vi "QScope.vi"() -> ()   [LabVIEW 2018]
uses:
  <vilib>/Utility/miscctls.llb/LVStringsAndValuesArrayTypeDef_DBL.ctl
  <vilib>/express/express signal manip/GetorSetDDTAttributes/Shared VIs/XDimension.ctl
  <vilib>/express/express signal manip/GetorSetDDTAttributes/Shared VIs/TimeType.ctl
  <vilib>/DAQmx/write.llb/DAQmx Write (Analog 1D DBL NChan 1Samp).vi
  <vilib>/DAQmx/read.llb/DAQmx Read (Analog 2D DBL NChan NSamp).vi
  <vilib>/DAQmx/miscellaneous.llb/DAQmx Fill In Error Info.vi
  <vilib>/express/express shared/transition.llb/Dynamic To Waveform Array.vi
  <vilib>/express/express signal manip/GetorSetDDTAttributes/Shared VIs/XDimension Enum to String.vi
  <vilib>/express/express signal manip/GetorSetDDTAttributes/Shared VIs/TimeMode Enum to Boolean.vi
  <vilib>/express/express signal manip/GetorSetDDTAttributes/Set DDT Attributes/SetT0.vi
  <vilib>/express/express signal manip/GetorSetDDTAttributes/Set DDT Attributes/sub Set StartTimeStamp.vi
  <vilib>/express/express shared/transition.llb/Waveform Array To Dynamic.vi
  <vilib>/express/express signal manip/GetorSetDDTAttributes/Get DDT Attributes/Get DDT Properties.xnode
  <vilib>/express/express signal manip/GetorSetDDTAttributes/Set DDT Attributes/Set DDT Properties.xnode
  <resource>/objmgr/daqmx.rc
  <vilib>/express/express signal manip/GetorSetDDTAttributes/Shared VIs/GetSetShared.lvlib
  <vilib>/express/express signal manip/GetorSetDDTAttributes/Set DDT Attributes/Set DDT Attributes.lvlib
panel:
  in  "trace display":enum32{"Time traces", "I-V plot", "Spectrum"}(tab)
  in  "Show \nrecord":i32 min=-1
  out "data":dbl[](graph) caption="Short Trace"
  out "data 2":dbl[](graph) caption="Full Trace"
  in  "Time slide":cluster{dbl, dbl}(slide) scale=0.0..100.0 scale format="%#_3g%"
  in  "short Channel":i8(ring) caption="Channel" items=["Dev2/ai0"]
  in  "long Channel":i8(ring) caption="Channel" items=["Dev2/ai0"]
  in  "fitting\nmethod":i32(ring)=1 items=["nearest", "linear", "spline"]
  out "Record\nTime":string caption="Comment"
  in  "refresh xy-plot":bool caption="Refresh"
  in  "y-channel":u16(ring) items=["Dev2/ai0"]
  in  "x-channel":u16(ring) items=["Dev2/ai0"]
  out "XY Graph":cluster{dbl[], dbl[]}(graph)
  out "time trace":cluster{"X":dbl, "Y":dbl}[](graph)
  out "Frequency domain":cluster{"X":dbl, "Y":dbl}[](graph)
  out "Spectrum":dbl[][](graph)
  in  "File tab":enum32{"File Operations"}(tab)
  in  "Comment\n(25 chars)":string
  out "mean values":dbl[](array[numeric])
  in  "Save to Path":path
  out "Last #":i32
  in  "File name prefix":string="ExpRec-"
  in  "Set threshold?":bool
  in  "Threshold":dbl min=0.0 max=20.0 format="%#_6p"
  out "min values":dbl[](array[numeric])
  out "max values":dbl[](array[numeric])
  out "standard deviation":dbl[](array[numeric])
  in  "Record data":bool
  out "TimeStamp":timestamp format="%<%I:%M:%S %p %d/%m/%Y>T"
  out "file operation error status":errorcluster caption="error out"
  out "Saving Data":bool
  out "active?":bool
  in  "DAQ control":enum32{"DAQ operation", "Analog Output"}(tab)
  in  "Tab Control":enum32{"Input", "Output"}(tab)
  in  "Input Channel List":i32[](listbox)
  in  "Term. Config.":i32(ring)=10083 items=["default"=-1, "RSE"=10083, "NRSE"=10078, "Differential"=10106, "Pseudodifferential"=12529]
  in  "section (s)":dbl=0.1 min=0.1 max=0.6 step=0.1 format="%#.2f"
  in  "full len(s)":dbl=10.0 min=0.5 max=60.0 step=0.5
  in  "Sampling rate (Hz)":dbl=5000.0
  in  "Output Channel List":i32[](listbox)
  in  "output values":dbl[](array[numeric]) format="%0.2f"
  in  "Init Channels":bool
  in  "stop":bool
  out "Recording in progress":bool
  in  "quit":bool
  out "mainloop error status":errorcluster
  out "DAQ error status":errorcluster
  out "DAQTask":refnum<k21>[](array[refnum])
  # "QingLAB@ASU\nhttps://qinglab.physics.edu.asu"
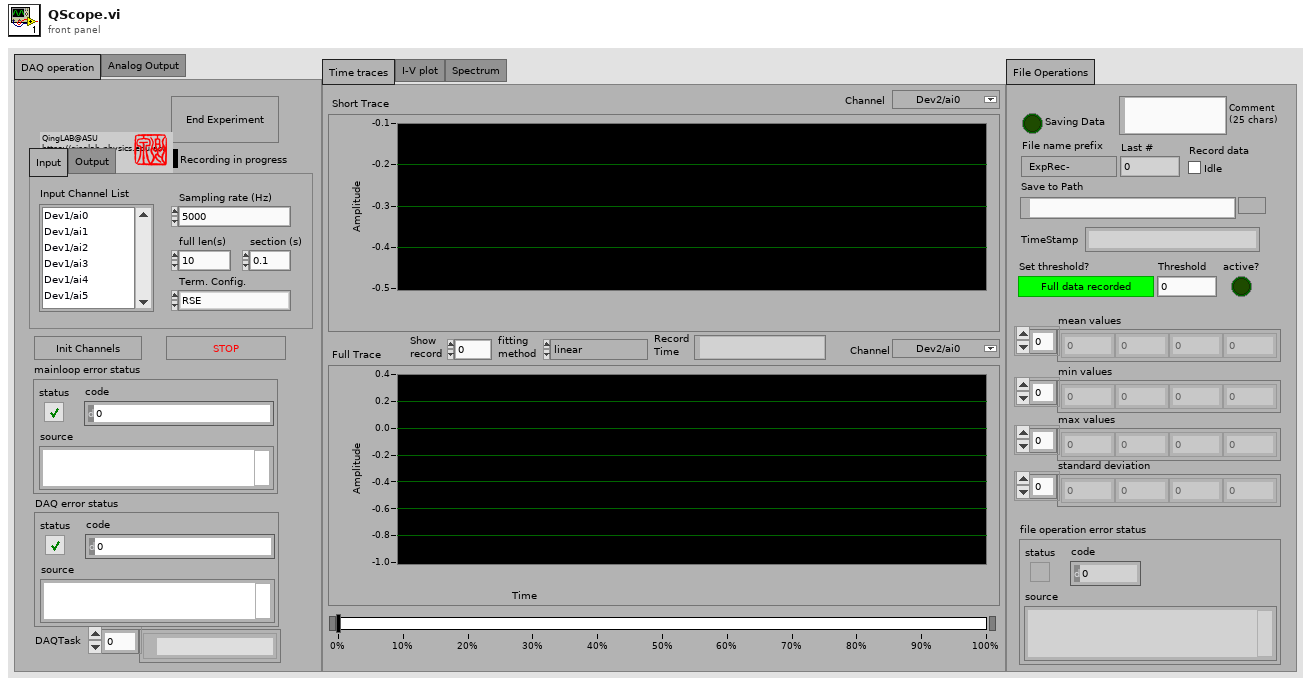
[diagram p1: front panel]
types:
  T1 = enum8{"Enabled", "Disabled", "Disabled and Grayed Out"}
  T2 = typedef "LVStringsAndValuesArrayTypeDef_DBL.ctl" = cluster{"String":string, "Value":dbl}[]
  T3 = cluster{i32, "task out":refnum<k21>[], "data":dbl[][]}
  T4 = typedef "GetSetShared.lvlib/TimeType.ctl" = enum16{"Absolute", "Relative"}
  T5 = typedef "GetSetShared.lvlib/XDimension.ctl" = enum16{"No Unit [-]", "Time [sec]", "Frequency [Hz]"}
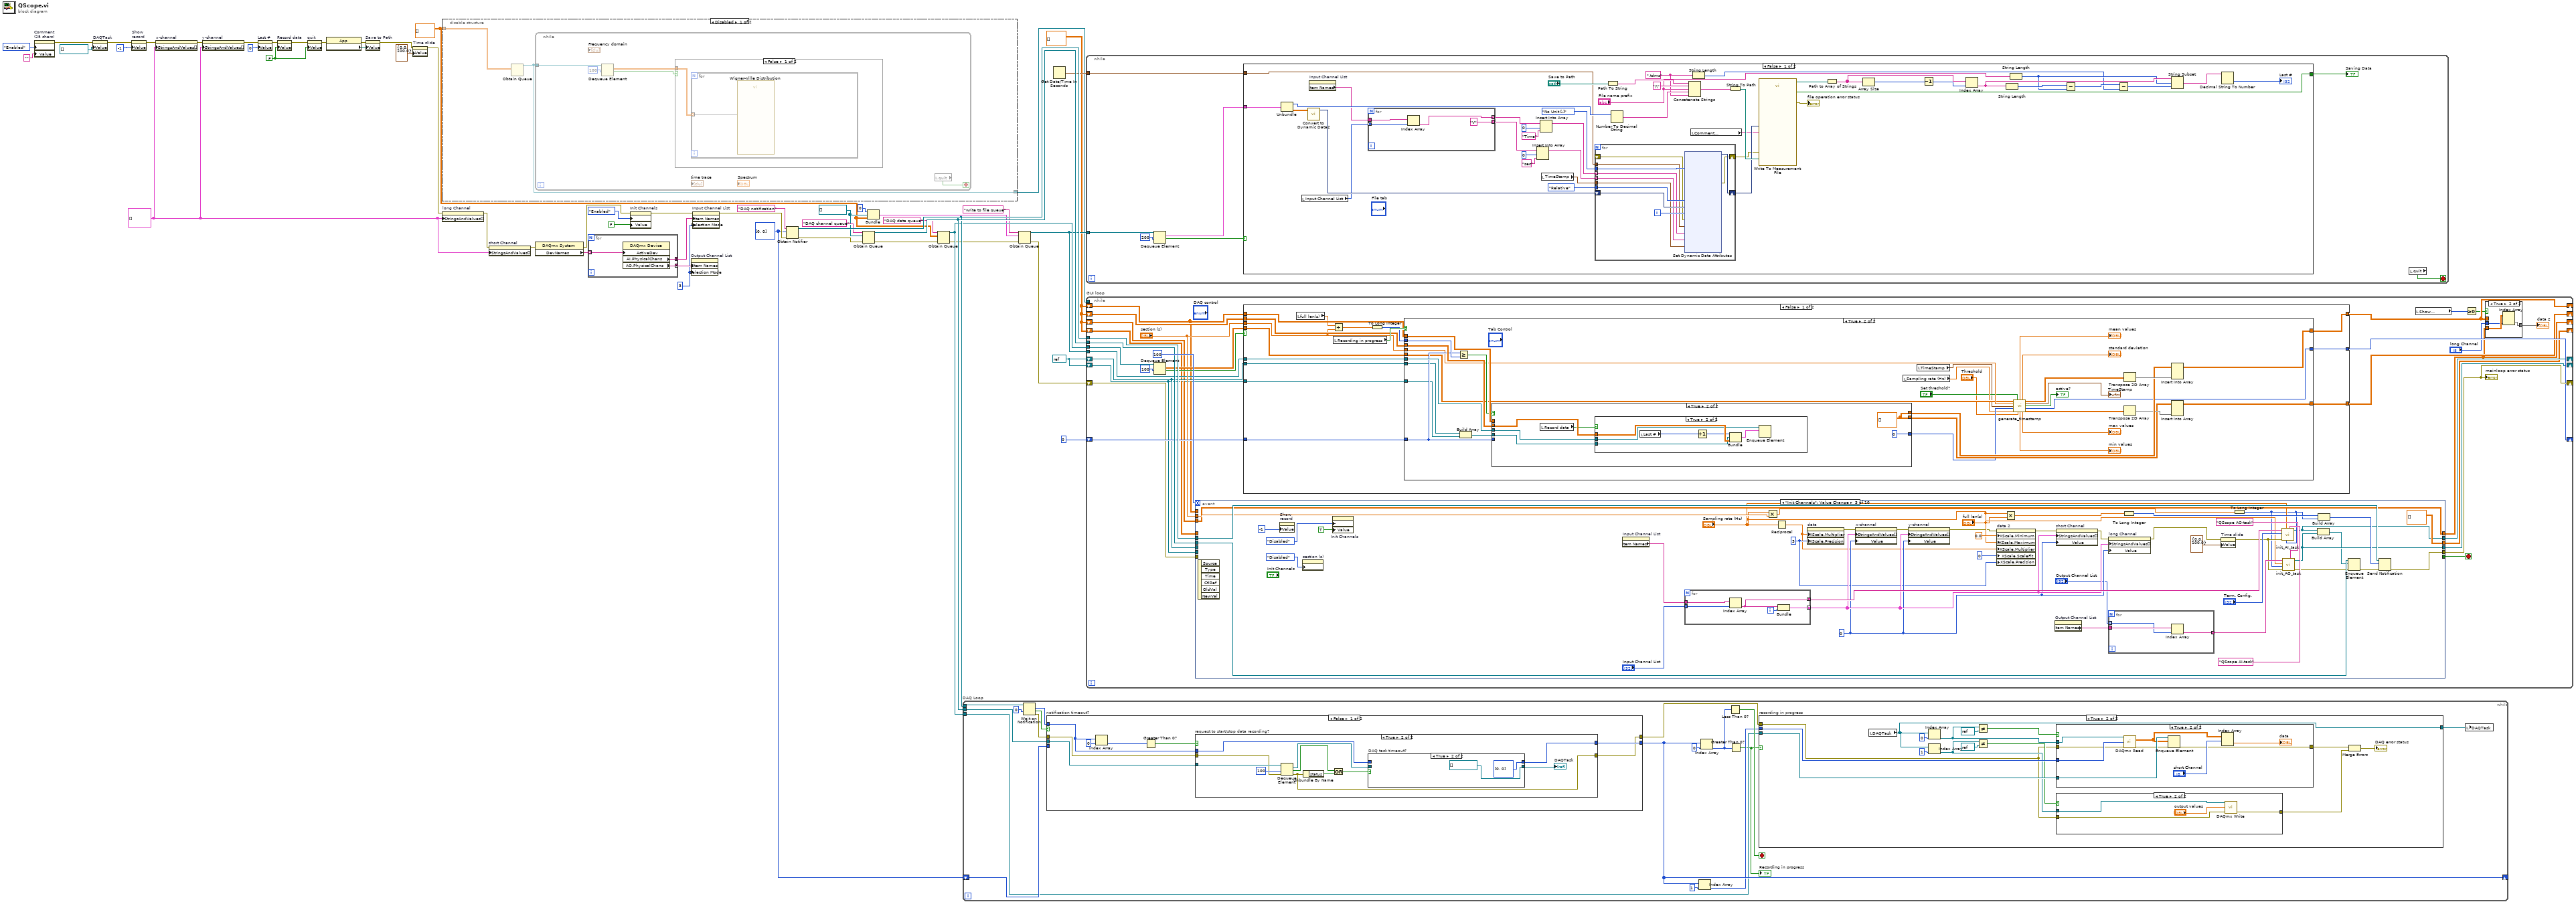
[diagram p0: block diagram]
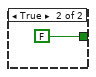
[diagram p4: hidden frame]
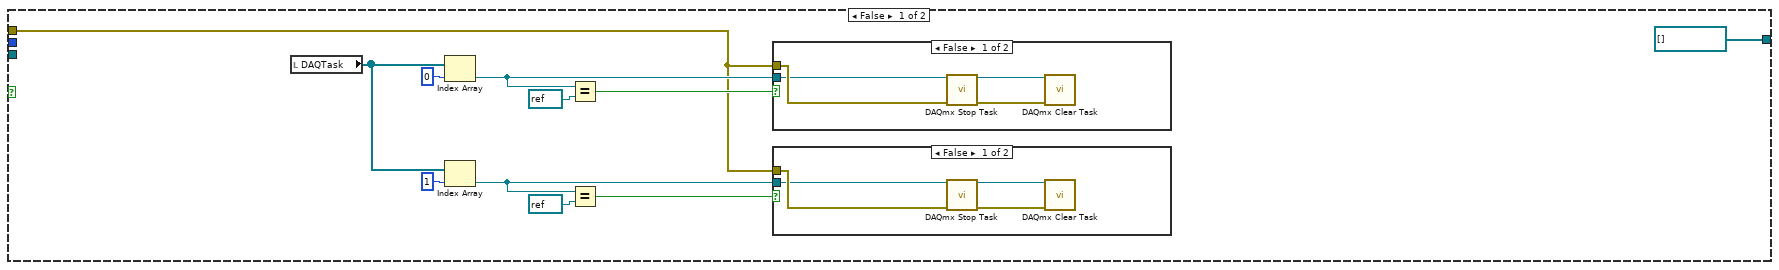
[diagram p5: hidden frame]
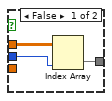
[diagram p13: hidden frame]
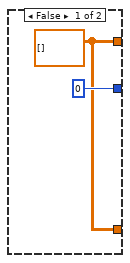
[diagram p14: hidden frame]
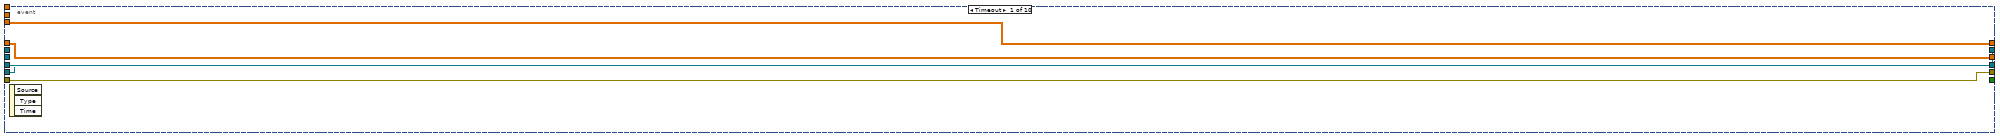
[diagram p18: hidden frame]
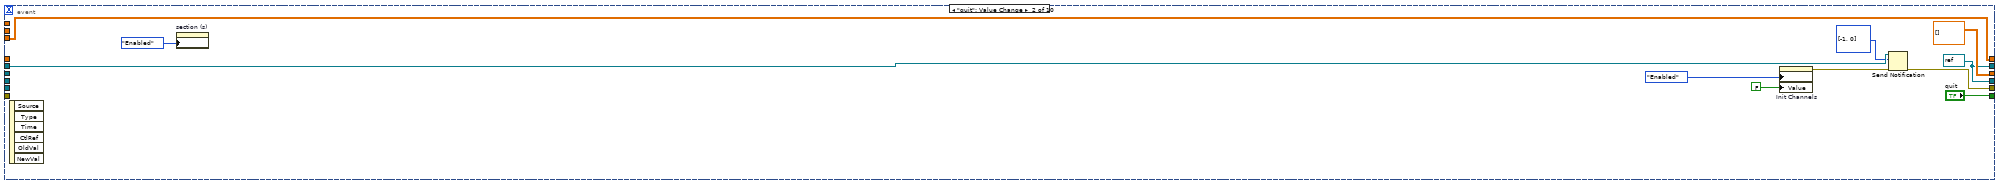
[diagram p19: hidden frame]
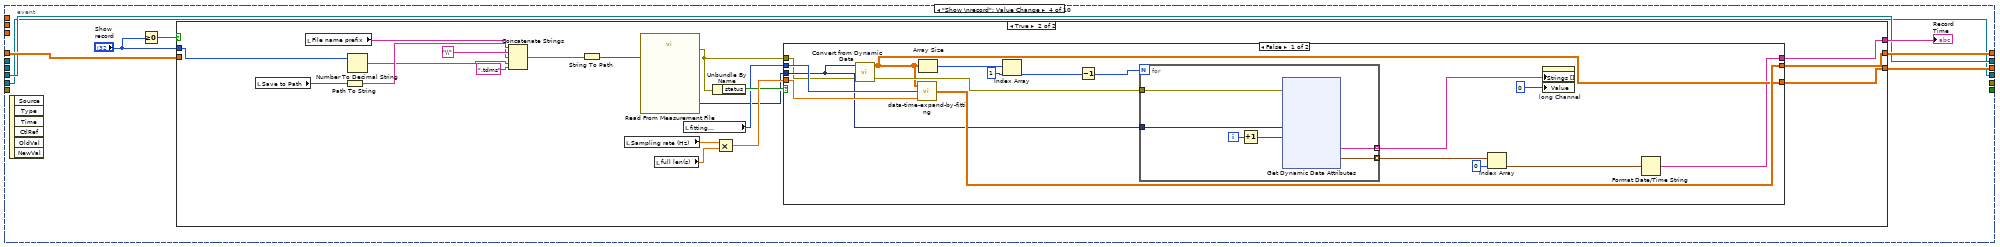
[diagram p20: hidden frame]
diagram:
  w21 = FALSE ("quit")
  w2 = refnum<k21> refnum ("task out")
  w10 = dbl[][] []
  w6 = dbl[][] [] ("data")
  w17 = T2 [] ("Strings And Values []")
  w44 = i32[] [0, 0]
  w25 = refnum<k21>[] [] ("task out")
  w3 = 3 ("Selection Mode")
  n1 = property on="Comment\n(25 chars)" class="Str"("DisabledEnum"=T1."Enabled" ("Disabled"), "Value"="" ("Comment\n(25 chars)")) -> (error out=w7:errorcluster)  [unwired: 2 in, 1 out]
  n2 = property on="DAQTask" class="Arr (strict)"(error in=w7, "Value"=refnum<k21>[] [] ("task out")) -> (error out=w11:errorcluster)  [unwired: 1 in, 1 out]
  n3 = property on="Show \nrecord" class="DigNum (strict)"(error in=w11, "Value"=-1 ("Show previous record")) -> (error out=w12:errorcluster)  [unwired: 1 in, 1 out]
  n4 = property on="x-channel" class="Ring (strict)"(error in=w12, "StringsAndValues[]"=w17) -> (error out=w16:errorcluster)  [unwired: 1 in, 1 out]
  n5 = property on="y-channel" class="Ring (strict)"(error in=w16, "StringsAndValues[]"=w17) -> (error out=w15:errorcluster)  [unwired: 1 in, 1 out]
  n6 = property on="Last #" class="DigNum (strict)"(error in=w15, "Value"=0 ("Last #")) -> (error out=w18:errorcluster)  [unwired: 1 in, 1 out]
  n7 = property on="Record data" class="Bool (strict)"(error in=w18, "Value"=w21) -> (error out=w20:errorcluster)  [unwired: 1 in, 1 out]
  n8 = property on="quit" class="Bool (strict)"(error in=w20, "Value"=w21) -> (error out=w22:errorcluster)  [unwired: 1 in, 1 out]
  n9 = property class="App"(error in=w22) -> (error out=w31:errorcluster, "App.DefaultDataLocation"=w32:path)  [unwired: 1 in, 1 out]
  n10 = property on="Save to Path" class="Path"(error in=w31, "Value"=w32) -> (error out=w30:errorcluster)  [unwired: 1 in, 1 out]
  n11 = property on="Time slide" class="Slide (strict)"(error in=w30, "Value"=cluster{dbl, dbl} {0.0, 100.0} ("Time slide")) -> (error out=w33:errorcluster)  [unwired: 1 in, 1 out]
  n12 = disable-structure shown="Disabled" {
    disable-tunnel: w6 -> [w55 _]
    disable-tunnel: [w54 _] -> w5
    frame Disabled {
      n13 = Obtain Queue(element data type=w55) -> (queue out=w54:refnum<queue>)  [unwired: 4 in, 2 out]
      n14 = while {
        tunnel: w54 -> [w59]
        stop <- w60 stop-if-true
        n15 = Dequeue Element(queue=w59, timeout in ms (-1)=100) -> (element=w56:dbl[][], timed out?=w57:bool)  [unwired: 1 in, 2 out]
        n16 = case shown="False" w57 {
          tunnel: w56 -> [w61 _]
          frame False {
            n17 = for {
              tunnel: w61 -> [w62] mode=indexing
              n18 = call "Wigner-Ville Distribution"("Signal"=w62) -> ()  [unwired: 6 in, 5 out]
            }
          }
          frame True {
          }
        }
        n19 = local read "quit"() -> (w60:bool)
      }
    }
    frame Enabled {
    }
  }
  n20 = property on="long Channel" class="Ring (strict)"(error in=w33, "StringsAndValues[]"=w17) -> (error out=w41:errorcluster)  [unwired: 1 in, 1 out]
  n21 = property on="short Channel" class="Ring (strict)"(error in=w41, "StringsAndValues[]"=w17) -> (error out=w42:errorcluster)  [unwired: 1 in, 1 out]
  n22 = property class="DAQmx System"(error in=w42) -> (error out=w43:errorcluster, "DevNames"=w53:tag[])  [unwired: 1 in, 1 out]
  n23 = for {
    tunnel: w53 -> [w65] mode=indexing
    tunnel: [w64] -> w52 mode=concatenating
    tunnel: [w63] -> w4 mode=concatenating
    n24 = property class="DAQmx Device"("ActiveDev"=w65) -> ("AI.PhysicalChans"=w64:tag[], "AO.PhysicalChans"=w63:tag[])  [unwired: 2 in, 2 out]
  }
  n25 = property on="Init Channels" class="Bool (strict)"(error in=w43, "DisabledEnum"=T1."Enabled" ("Disabled"), "Value"=FALSE ("Init Channels")) -> (error out=w46:errorcluster)  [unwired: 1 in, 1 out]
  n26 = property on="Output Channel List" class="LstBox (strict)"("Item Names"=w4, "Selection Mode"=w3) -> ()  [unwired: 2 in, 2 out]
  n27 = property on="Input Channel List" class="LstBox (strict)"(error in=w46, "Item Names"=w52, "Selection Mode"=w3) -> (error out=w47:errorcluster)  [unwired: 1 in, 1 out]
  n28 = Obtain Notifier(name (unnamed)="DAQ notification", notification data type=w44, error in (no error)=w47) -> (notifier out=w49:refnum<notifier>, error out=w48:errorcluster)  [unwired: 1 in, 1 out]
  n29 = Obtain Queue(name (unnamed)="DAQ channel queue", element data type=w25, error in (no error)=w48) -> (queue out=w50:refnum<queue>, error out=w37:errorcluster)  [unwired: 2 in, 1 out]
  n30 = Bundle(0, "task out"=w25, "data"=w6) -> (w24:T3)  [unwired: 1 in]
  n31 = Obtain Queue(name (unnamed)="DAQ data queue", element data type=w6, error in (no error)=w37) -> (queue out=w36:refnum<queue>, error out=w29:errorcluster)  [unwired: 2 in, 1 out]
  n32 = while "DAQ Loop" {
    tunnel: w50 -> [w78]
    tunnel: w49 -> [w81]
    shift-right: [w71] -> _
    shift-left: w44 -> [w76]
    tunnel: w36 -> [w69]
    stop <- w75 stop-if-true
    n33 = Wait on Notification(notifier=w81, timeout in ms (-1)=0) -> (notification=w79:i32[], timed out?=w80:bool, error out=w77:errorcluster)  [unwired: 2 in, 1 out]
    n34 = case "notification timeout?" shown="False" w80 {
      tunnel: w79 -> [w135 _]
      tunnel: w78 -> [w139 _]
      tunnel: w77 -> [w138 w157]
      tunnel: [w137 w158] -> w71
      tunnel: w76 -> [_ w158]
      tunnel: [w132 w157] -> w68
      frame False {
        n35 = Index Array(array=w135, index=0) -> (element=w133:i32)
        n36 = Greater Than 0?(x=w133) -> (x > 0?=w136:bool)
        n37 = case "request to start/stop data recording?" shown="True" w136 {
          tunnel: w139 -> [_ w152]
          tunnel: w138 -> [w140 w149]
          tunnel: [w141 w148] -> w137
          tunnel: w135 -> [w141 w147]
          tunnel: [w140 w146] -> w132
          frame False {
          }
          frame True {
            n38 = Dequeue Element(queue=w152, timeout in ms (-1)=100, error in (no error)=w149) -> (element=w150:refnum<k21>[], timed out?=w145:bool, error out=w146:errorcluster)  [unwired: 1 out]
            n39 = Unbundle By Name(w146) -> ("status"=w144:bool)
            n40 = Or(x=w145, y=w144) -> (x .or. y?=w143:bool)
            n41 = case "DAQ task timeout?" shown="True" w143 {
              tunnel: w150 -> [w154 _]
              tunnel: [w154 refnum<k21>[] [] ("task out")] -> w142
              tunnel: [w153 i32[] [0, 0]] -> w148
              tunnel: w147 -> [w153 _]
              frame False {
              }
              frame True {
              }
            }
            "DAQTask" <- w142
          }
        }
      }
      frame True {
      }
    }
    n42 = Index Array(array=w71, index=1) -> (element=w70:i32)
    n43 = Index Array(array=w71, index=0) -> (element=w73:i32)
    n44 = Less Than 0?(x=w73) -> (x < 0?=w75:bool)
    n45 = Greater Than 0?(x=w73) -> (x > 0?=w67:bool)
    "Recording in progress" <- w67
    n46 = case "recording in progress" shown="True" w67 {
      tunnel: w70 -> [_ w116]
      tunnel: w69 -> [_ w115]
      tunnel: w68 -> [w84 w106]
      tunnel: [refnum<k21>[] [] ("task out") w102] -> w66
      frame False {
        n47 = local read "DAQTask"() -> (w91:refnum<k21>[])
        n48 = Index Array(array=w91, index=0) -> (element=w88:refnum<k21>)
        n49 = Index Array(array=w91, index=1) -> (element=w85:refnum<k21>)
        n50 = Equal?(x=w88, y=refnum<k21> refnum ("task out")) -> (x = y?=w93:bool)
        n51 = Equal?(x=w85, y=refnum<k21> refnum ("task out")) -> (x = y?=w87:bool)
        n52 = case shown="False" w93 {
          tunnel: w84 -> [w99 _]
          tunnel: w88 -> [w98 _]
          frame False {
            n53 = call <vilib>:"DAQmx Stop Task.vi"("task/channels in"=w98, "error in"=w99) -> ("task out"=w101:refnum<k21>, "error out"=w100:errorcluster)  [unwired: 12 in]
            n54 = call <vilib>:"DAQmx Clear Task.vi"("task in"=w101, "error in"=w100) -> ()  [unwired: 13 in, 1 out]
          }
          frame True {
          }
        }
        n55 = case shown="False" w87 {
          tunnel: w84 -> [w95 _]
          tunnel: w85 -> [w94 _]
          frame False {
            n56 = call <vilib>:"DAQmx Stop Task.vi"("task/channels in"=w94, "error in"=w95) -> ("task out"=w97:refnum<k21>, "error out"=w96:errorcluster)  [unwired: 12 in]
            n57 = call <vilib>:"DAQmx Clear Task.vi"("task in"=w97, "error in"=w96) -> ()  [unwired: 13 in, 1 out]
          }
          frame True {
          }
        }
      }
      frame True {
        n58 = local read "DAQTask"() -> (w102:refnum<k21>[])
        n59 = Index Array(array=w102, index=0) -> (element=w111:refnum<k21>)
        n60 = Index Array(array=w102, index=1) -> (element=w107:refnum<k21>)
        n61 = Not Equal?(x=w111, y=refnum<k21> refnum) -> (x != y?=w113:bool)
        n62 = Not Equal?(x=w107, y=refnum<k21> refnum) -> (x != y?=w108:bool)
        n63 = case shown="True" w113 {
          tunnel: w116 -> [_ w131]
          tunnel: w115 -> [_ w128]
          tunnel: w106 -> [w122 w125]
          tunnel: w111 -> [_ w124]
          tunnel: [w122 w123] -> w105
          frame False {
          }
          frame True {
            n64 = call-poly <vilib>:"DAQmx Read.vi"("task/channels in"=w124, "number of samples per channel"=w131, "error in"=w125) -> ("data"=w127:dbl[][], "error out"=w126:errorcluster)  [unwired: 10 in, 1 out]
            n65 = Enqueue Element(queue=w128, element=w127, error in (no error)=w126) -> (error out=w123:errorcluster)  [unwired: 1 in, 2 out]
            n66 = Index Array(array=w127, index (row)="short Channel") -> (element=→"data":dbl[])  [unwired: 1 in]
          }
        }
        n67 = case shown="True" w108 {
          tunnel: w107 -> [_ w121]
          tunnel: w106 -> [w117 w119]
          tunnel: [w117 w118] -> w104
          frame False {
          }
          frame True {
            n68 = call-poly <vilib>:"DAQmx Write.vi"("task/channels in"=w121, "data"="output values", "error in"=w119) -> ("error out"=w118:errorcluster)  [unwired: 10 in, 2 out]
          }
        }
        n69 = Merge Errors(w105, w104) -> (→"DAQ error status":errorcluster)
      }
    }
    n70 = local write "DAQTask"(w66) -> ()
  }
  n71 = Obtain Queue(name (unnamed)="write to file queue", element data type=w24, error in (no error)=w29) -> (queue out=w26:refnum<queue>, error out=w28:errorcluster)  [unwired: 2 in, 1 out]
  n72 = Get Date/Time In Seconds() -> (seconds since 1Jan1904=w14:timestamp)
  n73 = while {
    tunnel: w26 -> [w165]
    tunnel: w14 -> [w160]
    stop <- w161 stop-if-true
    n74 = Dequeue Element(queue=w165, timeout in ms (-1)=200) -> (element=w162:T3, timed out?=w163:bool)  [unwired: 1 in, 2 out]
    n75 = case shown="False" w163 {
      tunnel: w162 -> [w208 _]
      tunnel: w160 -> [w168 _]
      tunnel: [w167 FALSE ("Saving Data")] -> w159
      frame False {
        w193 = ".tdms" ("string")
        n76 = Unbundle(w208) -> (w202:i32, "data"=w203:dbl[][])  [unwired: 1 out]
        n77 = local read "Input Channel List"() -> (w177:i32[])
        n78 = call "Convert to Dynamic Data2"("2D Array"=w203) -> ("Dynamic Data Type"=w184:dynamicdata)  [unwired: 3 in]
        n79 = property on="Input Channel List" class="LstBox (strict)"() -> ("Item Names"=w178:string[])  [unwired: 2 in, 2 out]
        n80 = for {
          tunnel: w178 -> [w212]
          tunnel: w177 -> [w211] mode=indexing
          tunnel: [w210] -> w176 mode=indexing
          tunnel: ["V"] -> w171 mode=indexing
          n81 = Index Array(array=w212, index=w211) -> (element=w210:string)
        }
        n82 = Insert Into Array(array=w171, index=0, new element="sec" ("new element/subarray")) -> (w169:string[])
        n83 = Insert Into Array(array=w176, index=0, new element="Time" ("new element/subarray")) -> (w170:string[])
        n84 = local read "TimeStamp"() -> (w183:timestamp)
        n85 = for {
          tunnel: w183 -> [w214]
          tunnel: XDimension."No Unit [-]" ("X Dimension") -> [w220]
          tunnel: TimeType."Relative" ("Time Mode") -> [w219]
          shift-right: [w222] -> w182
          shift-left: w184 -> [w223]
          shift-right: [w221] -> w181
          shift-left: _ -> [w217]
          tunnel: w170 -> [w216] mode=indexing
          tunnel: w169 -> [w215] mode=indexing
          tunnel: w168 -> [w213]
          i -> [w218]
          n86 = xnode "Set Dynamic Data Attributes"("Time Mode"=w219, "Signals In"=w223, "Signal Index"=w218, "error in"=w217, "Start Timestamp"=w213, "Signal Name"=w216, "Unit"=w215, "Timestamp"=w214, "X Dimension"=w220) -> ("Signals Out"=w222:dynamicdata, "error out"=w221:errorcluster)
        }
        n87 = Path To String(path="Save to Path") -> (string=w197:string)
        n88 = Number To Decimal String(number=w202) -> (decimal integer string=w196:string)  [unwired: 1 in]
        n89 = Concatenate Strings(w197, "\\" ("string"), "File name prefix", w196, w193) -> (w195:string)
        n90 = local read "Comment\n(25 chars)"() -> (w166:string)
        n91 = String Length(string=w193) -> (length=w188:i32)
        n92 = String To Path(string=w195) -> (path=w206:path)
        n93 = call "Write To Measurement File"("Signals"=w182, "error in (no error)"=w181, "Filename"=w206, "Comment"=w166) -> ("Filename Out"=w201:path, "Saving Data"=w167:bool, "error out"=→"file operation error status":errorcluster)  [unwired: 13 in]
        n94 = Path to Array of Strings(0:w201) -> (2:w200:string[])  [unwired: 1 out]
        n95 = Array Size(array=w200) -> (size(s)=w199:i32)
        n96 = Decrement(x=w199) -> (x-1=w198:i32)
        n97 = Index Array(array=w200, index=w198) -> (element=w192:string)
        n98 = String Length(string=w192) -> (length=w191:i32)
        n99 = String Length(string="File name prefix") -> (length=w190:i32)
        n100 = Subtract(x=w191, y=w190) -> (x-y=w189:i32)
        n101 = Subtract(x=w189, y=w188) -> (x-y=w187:i32)
        n102 = String Subset(string=w192, offset (0)=w190, length (rest)=w187) -> (substring=w186:string)
        n103 = Decimal String To Number(string=w186) -> (number=→"Last #":i32)  [unwired: 2 in, 1 out]
      }
      frame True {
      }
    }
    "Saving Data" <- w159
    n104 = local read "quit"() -> (w161:bool)
  }
  n105 = while "GUI loop" {
    tunnel: w50 -> [w286]
    tunnel: w49 -> [w285]
    shift-right: [w284] -> _
    shift-left: w28 -> [w268]
    tunnel: w36 -> [w283]
    shift-right: [w278] -> _
    shift-left: 0 -> [w279]
    shift-right: [w277] -> _
    shift-left: w10 -> [w269]
    shift-right: [w274] -> _
    shift-left: w10 -> [w270]
    shift-right: [w273] -> _
    shift-left: w2 -> [w272]
    tunnel: w26 -> [w271]
    shift-right: [w264] -> _
    shift-left: w10 -> [w267]
    shift-right: [w263] -> _
    shift-left: w10 -> [w262]
    tunnel: w5 -> [_]
    shift-right: [w260] -> _
    shift-left: w2 -> [w259]
    stop <- w287 stop-if-true
    n106 = Dequeue Element(queue=w283, timeout in ms (-1)=100) -> (element=w280:dbl[][], timed out?=w281:bool)  [unwired: 1 in, 2 out]
    n107 = event shown="[2] \"Init Channels\": Value Change" {
      selector: _ -> [_ _ _ _ _ _ _ _ _ _]
      dyn-events: _ -> [_ _ _ _ _ _ _ _ _ _]
      timeout: 100 -> [_ _ _ _ _ _ _ _ _ _]
      tunnel: [_ "quit" _ _ _ _ _ _ _ _] -> w287
      tunnel: w286 -> [_ _ w417 _ _ _ _ _ _ _]
      tunnel: w285 -> [_ w376 w416 _ _ _ _ _ _ w613]
      tunnel: [w364 w375 w414 _ _ _ _ _ _ w611] -> w284
      tunnel: "section (s)" -> [_ _ w408 _ _ _ _ _ _ _]
      tunnel: [w365 w366 w378 w431 w504 w511 w524 w542 w581 w601] -> w273
      tunnel: w272 -> [w365 _ _ w431 w504 w511 w524 w542 w581 _]
      tunnel: w269 -> [_ _ _ _ _ _ _ _ w584 _]
      tunnel: w268 -> [w364 _ _ _ _ _ _ _ _ _]
      tunnel: [w363 w368 w392 w435 w505 w518 w530 w541 w585 w603] -> w264
      tunnel: w267 -> [w363 w368 w392 _ w505 w518 _ w541 w585 w603]
      tunnel: [w362 dbl[][] [] ("Array") dbl[][] [] ("Array") w434 w506 w519 w529 w540 w582 dbl[][] [] ("Array")] -> w263
      tunnel: w262 -> [w362 _ _ w433 w506 w519 w529 w540 w582 _]
      tunnel: [w361 w366 w379 w430 w503 w512 w525 w539 w580 w601] -> w260
      tunnel: w259 -> [w361 _ _ w430 w503 w512 w525 w539 w580 _]
      event Timeout {
        n108 = event-data() -> ()  [unwired: 1 in, 3 out]
      }
      event "quit": Value Change {
        w366 = refnum<k21> refnum ("task out")
        n109 = event-data() -> ()  [unwired: 1 in, 6 out]
        n110 = property on="section (s)" class="DigNum (strict)"("DisabledEnum"=T1."Enabled" ("Disabled")) -> ()  [unwired: 2 in, 2 out]
        n111 = property on="Init Channels" class="Bool (strict)"("DisabledEnum"=T1."Enabled" ("Disabled"), "Value"=FALSE ("Init Channels")) -> (error out=w370:errorcluster)  [unwired: 2 in, 1 out]
        n112 = Send Notification(notification=i32[] [-1, 0], notifier=w376, error in (no error)=w370) -> (error out=w375:errorcluster)  [unwired: 1 out]
      }
      event "Init Channels": Value Change {
        w394 = u8 3 ("X Scale.Display Format:Precision")
        w396 = i8 0
        n113 = event-data() -> ()  [unwired: 1 in, 6 out]
        n114 = property on="Show \nrecord" class="DigNum (strict)"("Value"=-1 ("Show previous record")) -> ()  [unwired: 2 in, 2 out]
        n115 = property on="section (s)" class="DigNum (strict)"("DisabledEnum"=T1."Disabled" ("Disabled")) -> ()  [unwired: 2 in, 2 out]
        n116 = property on="Init Channels" class="Bool (strict)"("DisabledEnum"=T1."Disabled" ("Disabled"), "Value"=TRUE ("Value (Signaling)")) -> ()  [unwired: 2 in, 2 out]
        n117 = property on="Input Channel List" class="LstBox (strict)"() -> ("Item Names"=w409:string[])  [unwired: 2 in, 2 out]
        n118 = for {
          tunnel: "Input Channel List" -> [w429] mode=indexing
          tunnel: w409 -> [w428]
          tunnel: [w427] -> w411 mode=indexing
          tunnel: [w425] -> w399 mode=indexing
          i -> [w426]
          n119 = Index Array(array=w428, index=w429) -> (element=w427:string)
          n120 = Bundle(w427, w426) -> (w425:cluster{string, i32})  [unwired: 1 in]
        }
        n121 = Multiply(x="Sampling rate (Hz)", y=w408) -> (x*y=w413:dbl)
        n122 = Reciprocal(x="Sampling rate (Hz)") -> (1/x=w393:dbl)
        n123 = property on="data" class="WFGraph (strict)"("XScale.Multiplier"=w393, "XScale.Precision"=w394) -> (error out=w395:errorcluster)  [unwired: 2 in, 1 out]
        n124 = property on="x-channel" class="Ring (strict)"(error in=w395, "StringsAndValues[]"=w399, "Value"=w396) -> (error out=w398:errorcluster)  [unwired: 1 in, 1 out]
        n125 = property on="y-channel" class="Ring (strict)"(error in=w398, "StringsAndValues[]"=w399, "Value"=w396) -> (error out=w397:errorcluster)  [unwired: 1 in, 1 out]
        n126 = property on="data 2" class="WFGraph (strict)"(error in=w397, "XScale.Minimum"=0.0 ("X Scale.Range:Minimum"), "XScale.Maximum"="full len(s)", "XScale.Multiplier"=w393, "XScale.ScaleFit"=u8 0 ("X Scale.Scale Fit"), "XScale.Precision"=w394) -> (error out=w404:errorcluster)  [unwired: 1 in, 1 out]
        n127 = Multiply(x="Sampling rate (Hz)", y="full len(s)") -> (x*y=w418:dbl)
        n128 = property on="Output Channel List" class="LstBox (strict)"() -> ("Item Names"=w386:string[])  [unwired: 2 in, 2 out]
        n129 = property on="short Channel" class="Ring (strict)"(error in=w404, "StringsAndValues[]"=w399, "Value"=w396) -> (error out=w403:errorcluster)  [unwired: 1 in, 1 out]
        n130 = property on="long Channel" class="Ring (strict)"(error in=w403, "StringsAndValues[]"=w399, "Value"=w396) -> (error out=w402:errorcluster)  [unwired: 1 in, 1 out]
        n131 = for {
          tunnel: "Output Channel List" -> [w423] mode=indexing
          tunnel: w386 -> [w424]
          tunnel: [w422] -> w384 mode=indexing
          n132 = Index Array(array=w424, index=w423) -> (element=w422:string)
        }
        n133 = To Long Integer(number=w418) -> (32bit integer=w410:i32)
        n134 = property on="Time slide" class="Slide (strict)"(error in=w402, "Value"=cluster{dbl, dbl} {0.0, 100.0} ("Time slide")) -> (error out=w383:errorcluster)  [unwired: 1 in, 1 out]
        n135 = To Long Integer(number=w413) -> (32bit integer=w381:i32)
        n136 = call "init_AI_task.vi"("AI task name"="QScope AI-task", "number of samples"=w381, "rate"="Sampling rate (Hz)", "error in"=w383, "input terminal configuration"="Term. Config.", "AI channel list"=w411) -> ("task out"=w378:refnum<k21>)  [unwired: 4 in, 1 out]
        n137 = call "init_AO_task.vi"("new task name"="QScope AO-task", "error in"=w383, "samples per channel"=w381, "rate"="Sampling rate (Hz)", "AO channel list"=w384) -> ("error out"=w380:errorcluster, "task out"=w379:refnum<k21>)  [unwired: 5 in]
        n138 = Build Array(w378, w379) -> (w377:refnum<k21>[])
        n139 = Build Array(w410, w381) -> (w412:i32[])
        n140 = Enqueue Element(queue=w417, element=w377, error in (no error)=w380) -> (error out=w415:errorcluster)  [unwired: 1 in, 2 out]
        n141 = Send Notification(notification=w412, notifier=w416, error in (no error)=w415) -> (error out=w414:errorcluster)  [unwired: 1 out]
      }
      event "Show \nrecord": Value Change {
        n142 = event-data() -> ()  [unwired: 1 in, 6 out]
        n143 = Greater Or Equal To 0?(x="Show \nrecord") -> (x >= 0?=w437:bool)
        n144 = case shown="True" w437 {
          tunnel: "Show \nrecord" -> [_ w460]
          tunnel: [w442 w452] -> w435
          tunnel: [w442 w449] -> w434
          tunnel: w433 -> [_ _]
          tunnel: ["" ("date/time string") w446] -> w432
          frame False {
            w442 = dbl[][] [] ("yi")
            n145 = local read "Input Channel List"() -> (w440:i32[])
            n146 = property on="Input Channel List" class="LstBox (strict)"() -> ("Item Names"=w441:string[])  [unwired: 2 in, 2 out]
            n147 = for {
              tunnel: w441 -> [w445]
              tunnel: w440 -> [w444] mode=indexing
              tunnel: [w443] -> w439 mode=indexing
              n148 = Index Array(array=w445, index=w444) -> (element=w443:string)
            }
            n149 = property on="long Channel" class="Ring (strict)"("Strings []"=w439) -> ()  [unwired: 2 in, 2 out]
          }
          frame True {
            n150 = local read "Save to Path"() -> (w464:path)
            n151 = local read "File name prefix"() -> (w461:string)
            n152 = Path To String(path=w464) -> (string=w463:string)
            n153 = Number To Decimal String(number=w460) -> (decimal integer string=w459:string)  [unwired: 1 in]
            n154 = Concatenate Strings(w463, "\\" ("string"), w461, w459, ".tdms" ("string")) -> (w457:string)
            n155 = String To Path(string=w457) -> (path=w456:path)
            n156 = local read "Sampling rate (Hz)"() -> (w455:dbl)
            n157 = call "Read From Measurement File"("Filename"=w456) -> ("error out"=w447:errorcluster, "Signals"=w448:dynamicdata)  [unwired: 5 in, 4 out]
            n158 = local read "full len(s)"() -> (w454:dbl)
            n159 = local read "fitting\nmethod"() -> (w450:i32)
            n160 = Unbundle By Name(w447) -> ("status"=w451:bool)
            n161 = Multiply(x=w455, y=w454) -> (x*y=w453:dbl)
            n162 = case shown="False" w451 {
              tunnel: w453 -> [w479 _]
              tunnel: [w478 w502] -> w452
              tunnel: w450 -> [w480 _]
              tunnel: w448 -> [w477 _]
              tunnel: [w475 w502] -> w449
              tunnel: w447 -> [w476 _]
              tunnel: [w465 "" ("date/time string")] -> w446
              frame False {
                n163 = call "Convert from Dynamic Data"("Dynamic Data Type"=w477) -> ("Array"=w475:dbl[][])  [unwired: 3 in]
                n164 = call "data-time-expand-by-fitting.vi"("Num of Samples"=w479, "fitting\nmethod"=w480, "data in"=w475) -> ("data out"=w478:dbl[][])
                n165 = Array Size(array=w475) -> (size(s)=w474:i32[])
                n166 = Index Array(array=w474, index=1) -> (element=w473:i32)
                n167 = Decrement(x=w473) -> (x-1=w469:i32)
                n168 = for {
                  N: w469 -> [_]
                  tunnel: w477 -> [w486]
                  tunnel: w476 -> [w485]
                  tunnel: [w483] -> w472 mode=indexing
                  tunnel: [w481] -> w468 mode=indexing
                  i -> [w484]
                  n169 = Increment(x=w484) -> (x+1=w482:i32)
                  n170 = xnode "Get Dynamic Data Attributes"("Signals In"=w486, "Signal Index"=w482, "error in"=w485) -> ("Signal Name"=w483:string, "Timestamp"=w481:timestamp)  [unwired: 2 out]
                }
                n171 = Index Array(array=w468, index=0) -> (element=w466:timestamp)
                n172 = property on="long Channel" class="Ring (strict)"("Strings []"=w472, "Value"=i8 0) -> ()  [unwired: 2 in, 2 out]
                n173 = Format Date/Time String(seconds (now)=w466) -> (date/time string=w465:string)  [unwired: 2 in]
              }
              frame True {
                w502 = dbl[][] [] ("yi")
              }
            }
          }
        }
        "Record\nTime" <- w432
      }
      event "Record data": Value Change {
        n174 = event-data() -> ()  [unwired: 1 in, 6 out]
        n175 = case shown="True" "Record data" {
          frame False {
            n176 = property on="Comment\n(25 chars)" class="Str"("DisabledEnum"=T1."Enabled" ("Disabled"), "Value"="" ("Comment")) -> ()  [unwired: 2 in, 2 out]
          }
          frame True {
            n177 = property on="Comment\n(25 chars)" class="Str"("DisabledEnum"=T1."Disabled and Grayed Out" ("Disabled")) -> ()  [unwired: 2 in, 2 out]
          }
        }
      }
      event "Comment\n(25 chars)": Value Change {
        w514 = 25 ("y")
        n178 = event-data() -> ()  [unwired: 1 in, 1 out]
        n179 = String Length(string="Comment\n(25 chars)") -> (length=w517:i32)
        n180 = Greater?(x=w517, y=w514) -> (0:w516:bool)
        n181 = case shown="False" w516 {
          tunnel: "Comment\n(25 chars)" -> [w520 w523]
          tunnel: w514 -> [_ w522]
          tunnel: [w520 w521] -> w513
          frame False {
          }
          frame True {
            n182 = String Subset(string=w523, length (rest)=w522) -> (substring=w521:string)  [unwired: 1 in]
          }
        }
        n183 = local write "Comment\n(25 chars)"(w513) -> ()
      }
      event "fitting\nmethod": Value Change {
        n184 = event-data() -> ()  [unwired: 1 in, 6 out]
        n185 = local read "Sampling rate (Hz)"() -> (w528:dbl)
        n186 = local read "Show \nrecord"() -> (w533:i32)
        n187 = local read "full len(s)"() -> (w527:dbl)
        n188 = Multiply(x=w528, y=w527) -> (x*y=w526:dbl)
        n189 = Greater Or Equal To 0?(x=w533) -> (x >= 0?=w532:bool)
        n190 = case shown="True" w532 {
          tunnel: w529 -> [_ w537]
          tunnel: "fitting\nmethod" -> [_ w538]
          tunnel: [dbl[][] [] ("data out") w536] -> w530
          tunnel: w526 -> [_ w535]
          frame False {
          }
          frame True {
            n191 = call "data-time-expand-by-fitting.vi"("Num of Samples"=w535, "fitting\nmethod"=w538, "data in"=w537) -> ("data out"=w536:dbl[][])
          }
        }
      }
      event "Time slide": Value Change {
        w546 = 100.0 ("y")
        n192 = event-data() -> ()  [unwired: 1 in, 1 out]
        n193 = Unbundle("Time slide") -> (w558:dbl, w557:dbl)
        n194 = Equal?(x=w558, y=w557) -> (x = y?=w559:bool)
        n195 = case shown="True" w559 {
          tunnel: w558 -> [w566 w568]
          tunnel: w557 -> [w565 _]
          tunnel: [w566 w569] -> w555
          tunnel: [w565 w567] -> w554
          frame False {
          }
          frame True {
            n196 = Add(x=w568, y=1.0) -> (x+y=w572:dbl)
            n197 = Greater?(x=w572, y=100.0) -> (0:w570:bool)
            n198 = case shown="True" w570 {
              tunnel: w568 -> [w575 w579]
              tunnel: [w575 w576] -> w569
              tunnel: w568 -> [w574 w576]
              tunnel: [w574 w577] -> w567
              frame False {
              }
              frame True {
                n199 = Subtract(x=w579, y=1.0) -> (x-y=w577:dbl)
              }
            }
          }
        }
        n200 = Greater?(x=w555, y=w554) -> (0:w556:bool)
        n201 = case shown="True" w556 {
          tunnel: [w562 w564] -> w551
          tunnel: w555 -> [w561 w564]
          tunnel: w554 -> [w562 w563]
          tunnel: [w561 w563] -> w552
          frame False {
          }
          frame True {
          }
        }
        n202 = local read "full len(s)"() -> (w553:dbl)
        n203 = Multiply(x=w553, y=w552) -> (x*y=w548:dbl)
        n204 = Multiply(x=w553, y=w551) -> (x*y=w547:dbl)
        n205 = Bundle(w552, w551) -> (w550:cluster{dbl, dbl})  [unwired: 1 in]
        n206 = property on="Time slide" class="Slide (strict)"("Value"=w550) -> ()  [unwired: 2 in, 2 out]
        n207 = Divide(x=w548, y=w546) -> (x/y=w549:dbl)
        n208 = Divide(x=w547, y=w546) -> (x/y=w545:dbl)
        n209 = property on="data 2" class="WFGraph (strict)"("XScale.Minimum"=w549, "XScale.Maximum"=w545, "XScale.ScaleFit"=u8 0 ("X Scale.Scale Fit"), "XScale.Precision"=u8 3 ("X Scale.Display Format:Precision")) -> ()  [unwired: 2 in, 2 out]
      }
      event "trace display", "x-channel", "y-channel", "refresh xy-plot": Value Change {
        n210 = event-data() -> ()  [unwired: 1 in, 6 out]
        n211 = local read "Show \nrecord"() -> (w587:i32)
        n212 = Greater Or Equal To 0?(x=w587) -> (x >= 0?=w586:bool)
        n213 = case shown="False" w586 {
          tunnel: w585 -> [_ w590]
          tunnel: [w589 w590] -> w583
          tunnel: w584 -> [w589 _]
          frame False {
          }
          frame True {
          }
        }
        n214 = case shown="\"I-V plot\"" "trace display" {
          tunnel: w583 -> [_ w600]
          frame "Time traces", Default {
          }
          frame "I-V plot" {
            n215 = property on="x-channel" class="Ring (strict)"() -> ("Strings []"=w596:string[])  [unwired: 2 in, 2 out]
            n216 = property on="y-channel" class="Ring (strict)"() -> ("Strings []"=w594:string[])  [unwired: 2 in, 2 out]
            n217 = Index Array(array=w600, index (col)="x-channel") -> (element=w599:dbl[])  [unwired: 1 in]
            n218 = Index Array(array=w600, index (col)="y-channel") -> (element=w598:dbl[])  [unwired: 1 in]
            n219 = Index Array(array=w596, index="x-channel") -> (element=w595:string)
            n220 = Index Array(array=w594, index="y-channel") -> (element=w593:string)
            n221 = property on="XY Graph" class="XYGraph (strict)"("XScale.NameLbl.Text"=w595, "YScale.NameLbl.Text"=w593) -> ()  [unwired: 2 in, 2 out]
            n222 = Bundle(w599, w598) -> (→"XY Graph":cluster{dbl[], dbl[]})  [unwired: 1 in]
          }
        }
      }
      event "stop": Value Change {
        w601 = refnum<k21> refnum ("task out")
        w604 = T2 [] ("Strings And Values []")
        n223 = event-data() -> ()  [unwired: 1 in, 6 out]
        n224 = property on="section (s)" class="DigNum (strict)"("DisabledEnum"=T1."Enabled" ("Disabled")) -> ()  [unwired: 2 in, 2 out]
        n225 = property on="y-channel" class="Ring (strict)"("StringsAndValues[]"=w604) -> (error out=w606:errorcluster)  [unwired: 2 in, 1 out]
        n226 = property on="x-channel" class="Ring (strict)"(error in=w606, "StringsAndValues[]"=w604) -> (error out=w605:errorcluster)  [unwired: 1 in, 1 out]
        n227 = property on="long Channel" class="Ring (strict)"(error in=w605, "StringsAndValues[]"=w604) -> (error out=w610:errorcluster)  [unwired: 1 in, 1 out]
        n228 = property on="short Channel" class="Ring (strict)"(error in=w610, "StringsAndValues[]"=w604) -> (error out=w609:errorcluster)  [unwired: 1 in, 1 out]
        n229 = Send Notification(notification=i32[] [0, 0], notifier=w613, error in (no error)=w609) -> (error out=w612:errorcluster)  [unwired: 1 out]
        n230 = property on="Init Channels" class="Bool (strict)"(error in=w612, "DisabledEnum"=T1."Enabled" ("Disabled"), "Value"=FALSE ("Init Channels")) -> (error out=w611:errorcluster)  [unwired: 1 in, 1 out]
      }
    }
    "mainloop error status" <- w284
    n231 = case shown="False" w281 {
      tunnel: w280 -> [w302 _]
      tunnel: w279 -> [w307 w360]
      tunnel: [w301 w360] -> w278
      tunnel: w269 -> [w308 w359]
      tunnel: [w306 w359] -> w277
      tunnel: "section (s)" -> [w296 _]
      tunnel: w270 -> [w300 w358]
      tunnel: [w299 w358] -> w274
      tunnel: w272 -> [w298 _]
      tunnel: w271 -> [w297 _]
      tunnel: w259 -> [w295 _]
      frame False {
        n232 = local read "full len(s)"() -> (w305:dbl)
        n233 = Divide(x=w305, y=w296) -> (x/y=w304:dbl)
        n234 = local read "Recording in progress"() -> (w309:bool)
        n235 = To Long Integer(number=w304) -> (32bit integer=w303:i32)
        n236 = case shown="True" w309 {
          tunnel: [0 w329] -> w301
          tunnel: w302 -> [_ w327]
          tunnel: w308 -> [_ w340]
          tunnel: w307 -> [_ w331]
          tunnel: [w310 w342] -> w306
          tunnel: w303 -> [_ w333]
          tunnel: w300 -> [_ w336]
          tunnel: [w310 w337] -> w299
          tunnel: w298 -> [_ w314]
          tunnel: w297 -> [_ w334]
          tunnel: w296 -> [_ w328]
          tunnel: w295 -> [_ w313]
          frame False {
            w310 = dbl[][] []
          }
          frame True {
            n237 = Greater Or Equal?(x=w331, y=w333) -> (x >= y?=w332:bool)
            n238 = Build Array(w314, w313) -> (w312:refnum<k21>[])
            n239 = case shown="True" w332 {
              tunnel: [w343 0] -> w330
              tunnel: w340 -> [w345 _]
              tunnel: [w345 w350] -> w339
              tunnel: w336 -> [w344 w349]
              tunnel: [w344 w350] -> w335
              tunnel: w334 -> [_ w348]
              tunnel: w331 -> [w343 _]
              tunnel: w312 -> [_ w346]
              frame False {
              }
              frame True {
                w350 = dbl[][] []
                n240 = local read "Record data"() -> (w347:bool)
                n241 = case shown="True" w347 {
                  tunnel: w349 -> [_ w357]
                  tunnel: w348 -> [_ w356]
                  tunnel: w346 -> [_ w353]
                  frame False {
                  }
                  frame True {
                    n242 = local read "Last #"() -> (w355:i32)
                    n243 = Increment(x=w355) -> (x+1=w354:i32)
                    n244 = Bundle(w354, w353, w357) -> (w352:cluster{i32, refnum<k21>[], dbl[][]})  [unwired: 1 in]
                    n245 = Enqueue Element(queue=w356, element=w352) -> ()  [unwired: 2 in, 3 out]
                  }
                }
              }
            }
            n246 = local read "Sampling rate (Hz)"() -> (w326:dbl)
            n247 = local read "TimeStamp"() -> (w315:timestamp)
            n248 = call "generate_timestamp.vi"("data in"=w327, "Set threshold on standard deviation"="Set threshold?", "interval time (s)"=w328, "time stamp in"=w315, "index in"=w330, "Sampling rate (Hz)"=w326, "Threshold of standard deviation"="Threshold") -> ("mean values"=→"mean values":dbl[], "standard deviation"=→"standard deviation":dbl[], "data out"=w317:dbl[][], "time stamp out"=→"TimeStamp":timestamp, "data averaged"=→"active?":bool, "index out"=w329:i32, "min values"=→"min values":dbl[], "max values"=→"max values":dbl[], "data with time"=w318:dbl[][])
            n249 = Transpose 2D Array(2D array=w317) -> (transposed array=w341:dbl[][])
            n250 = Transpose 2D Array(2D array=w318) -> (transposed array=w338:dbl[][])
            n251 = Insert Into Array(array=w339, new element=w341) -> (w342:dbl[][])  [unwired: 2 in]
            n252 = Insert Into Array(array=w335, new element=w338) -> (w337:dbl[][])  [unwired: 2 in]
          }
        }
      }
      frame True {
      }
    }
    n253 = local read "Show \nrecord"() -> (w266:i32)
    n254 = Greater Or Equal To 0?(x=w266) -> (x >= 0?=w265:bool)
    n255 = case shown="True" w265 {
      tunnel: w277 -> [w291 _]
      tunnel: "long Channel" -> [w290 w293]
      tunnel: w264 -> [_ w294]
      tunnel: [w289 w292] -> w261
      frame False {
        n256 = Index Array(array=w291, index (col)=w290) -> (element=w289:dbl[])  [unwired: 1 in]
      }
      frame True {
        n257 = Index Array(array=w294, index (col)=w293) -> (element=w292:dbl[])  [unwired: 1 in]
      }
    }
    "data 2" <- w261
  }
